vi "Main.vi"(11 "Module Admin":refnum<class "Delacor_lib_QMH_Module Admin.lvclass">) -> ()   [LabVIEW 2026, in "Servo Motor Emulator.lvlib"]
doc: "This template is based off of the Queued Message Handler design pattern and the Queued Message Handler project template that ships with LabVIEW.\n\nThe main difference is that the queue is private to this module and communication between modules is performed via Broadcast and Request events.\n\nRequest events are wrapped in public API methods and are handled in the Event Handling Loop (EHL) of this VI. Any module can register for Broadcast events sent by this module. The EHL generates messages based on user interface actions.\n\nThe Message Handling Loop (MHL) processes messages generated by the EHL, or by other messages. The messages are string values, so new messages can be added easily to the Message Cases case structure in the MHL. Each message cluster can also provide an optional value for Message Data, which is a variant that can be converted to whatever message-specific data is required.\n_____\nBased on DQMH Dev Tools: Project Template 7.1.2.1547."
uses:
  Servo Motor Emulator.lvlib
  <vilib>/Delacor/Delacor QMH/Libraries/Module Admin_class/Delacor_lib_QMH_Module Admin.lvclass
  Module Data--cluster.ctl
  Stop Argument--cluster.ctl
  <vilib>/Delacor/Delacor QMH/Libraries/Message Queue_class/Delacor_lib_QMH_Message Queue.lvclass/Delacor_lib_QMH_Message Queue.ctl
  <vilib>/Delacor/Delacor QMH/Libraries/Module Admin_class/Delacor_lib_QMH_Module Admin.lvclass/Delacor_lib_QMH_Module Admin.ctl
  Update Position Argument--cluster.ctl
  <vilib>/Utility/miscctls.llb/LVPointTypeDef.ctl
  <vilib>/Delacor/Delacor QMH/Libraries/Message Queue_class/Delacor_lib_QMH_Enqueue Message (Single).vi
  <vilib>/Delacor/Delacor QMH/Libraries/Module Admin_class/Delacor_lib_QMH_Get External Launch.vi
  <vilib>/Delacor/Delacor QMH/Libraries/Message Queue_class/Delacor_lib_QMH_Message Queue.lvclass
panel:
  in  "RH":dbl
  in  "Temperature":dbl
  out "Position":dbl(knob) scale=0.0..180.0
  out "error out":errorcluster
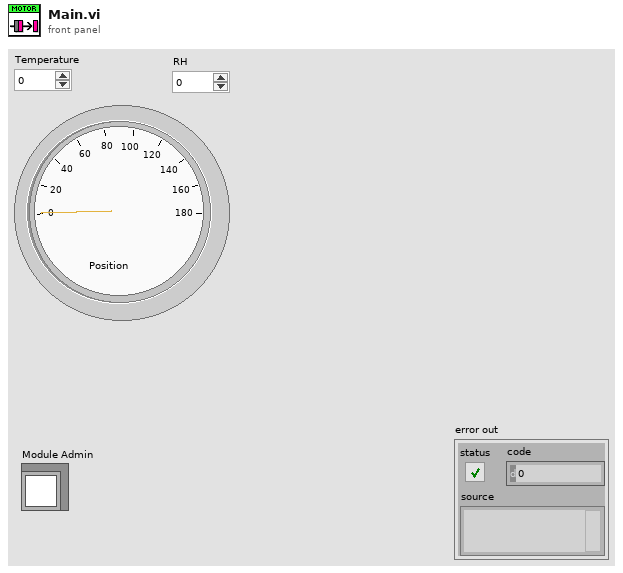
[diagram p1: front panel]
types:
  T1 = typedef "Servo Motor Emulator.lvlib/Request Events--cluster.ctl" = cluster{"Stop Module":refnum<user-event>, "Show Panel":refnum<user-event>, "Hide Panel":refnum<user-event>, "Get Module Execution Status":refnum<user-event>, "Show Diagram":refnum<user-event>, "Update Position":refnum<user-event>}
  T2 = typedef "Servo Motor Emulator.lvlib/Module Data--cluster.ctl" = cluster{"Status":string}
  T3 = enum32{"invalid lock state", "Not Locked", "Locked (No Password)", "Password-protected"}
  T4 = typedef "Servo Motor Emulator.lvlib/Stop Argument--cluster.ctl" = cluster{"Origin":string, "Exit via Stop Module Req?":bool, "Wait for Module to stop?":bool}
  T5 = typedef "Servo Motor Emulator.lvlib/Update Position Argument--cluster.ctl" = cluster{"Position":dbl}
  T6 = typedef "LVPointTypeDef.ctl" = cluster{"Horizontal":i16, "Vertical":i16}
  T7 = enum32{"Invalid", "Standard", "Closed", "Hidden", "Minimized", "Maximized"}
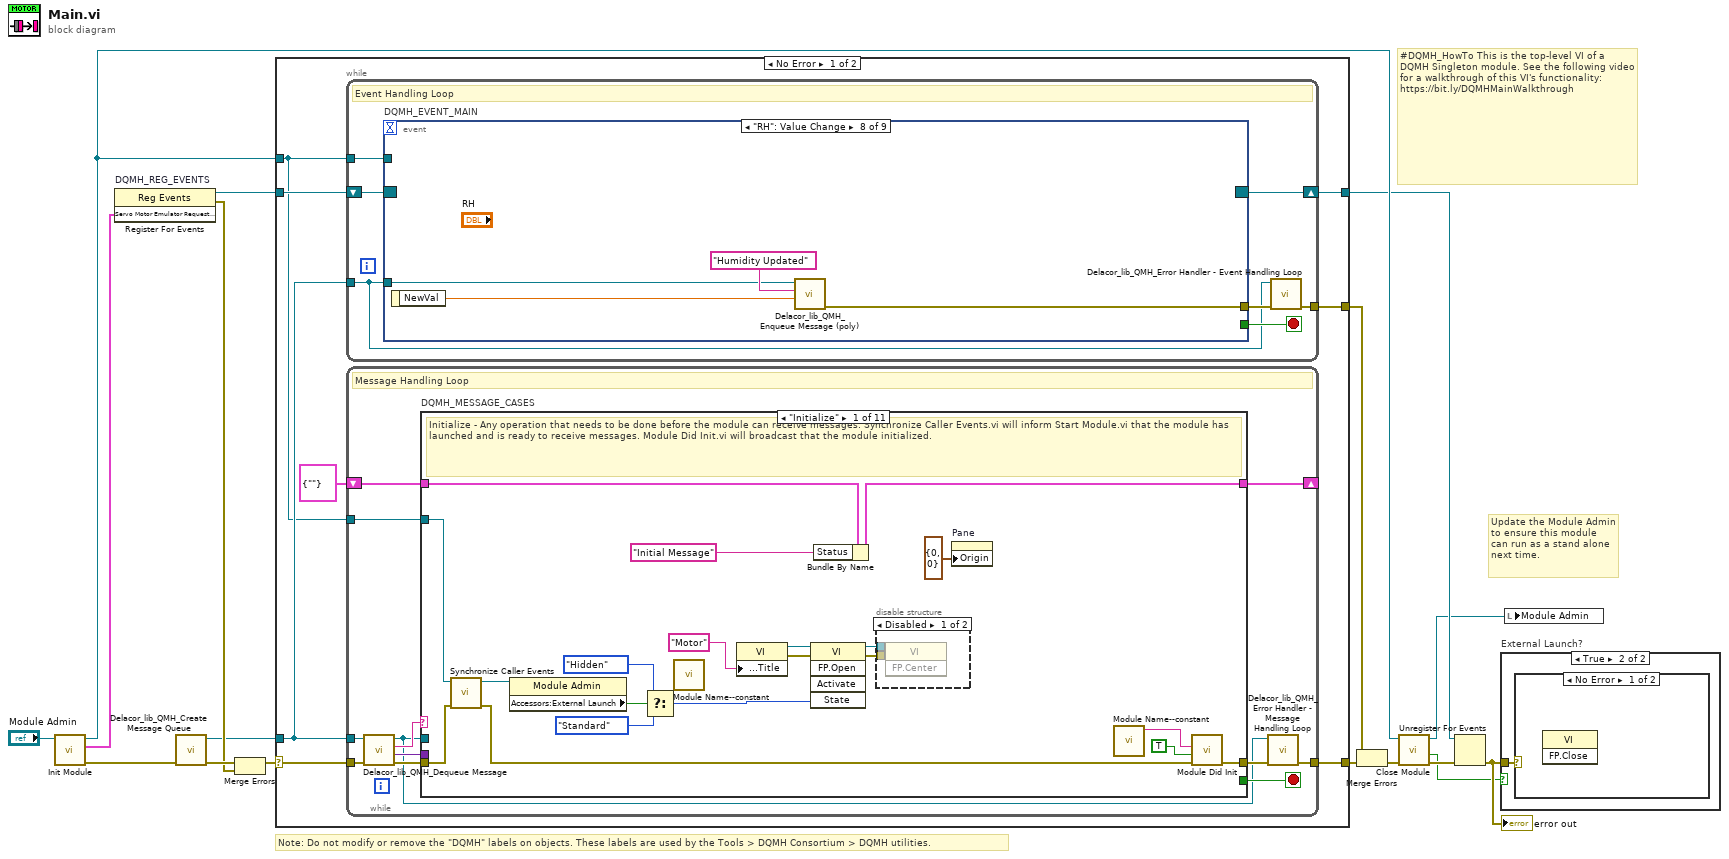
[diagram p0: block diagram]
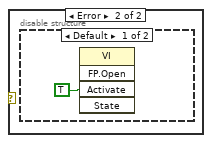
[diagram p3: hidden frame]
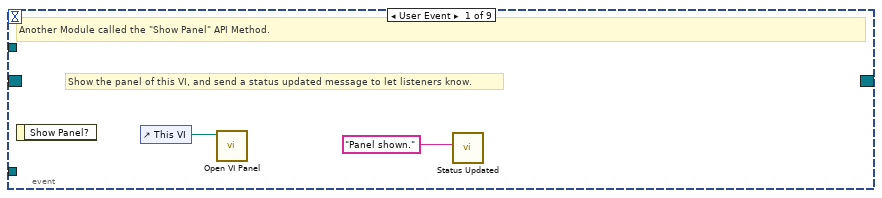
[diagram p5: hidden frame]
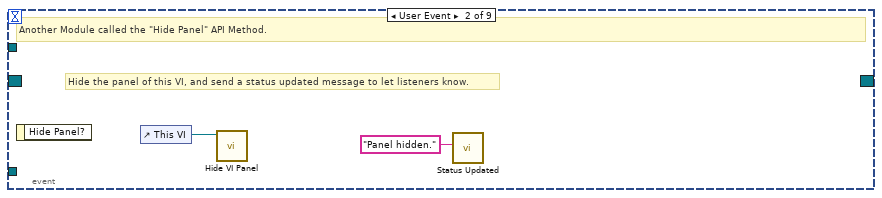
[diagram p6: hidden frame]
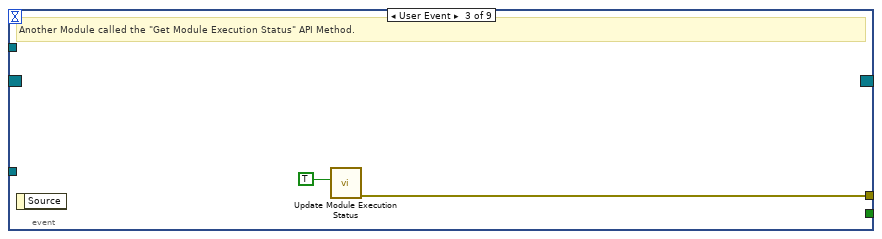
[diagram p7: hidden frame]
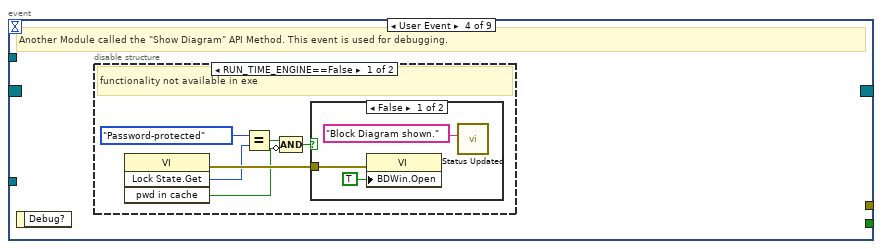
[diagram p8: hidden frame]
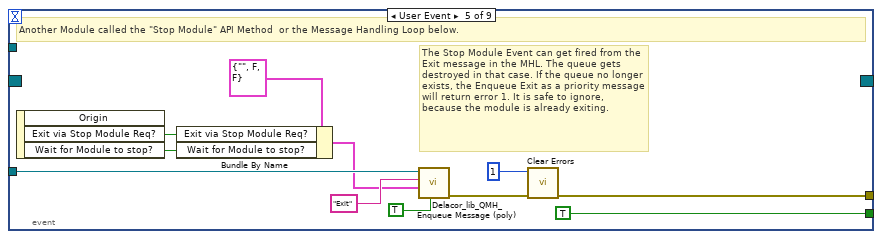
[diagram p11: hidden frame]
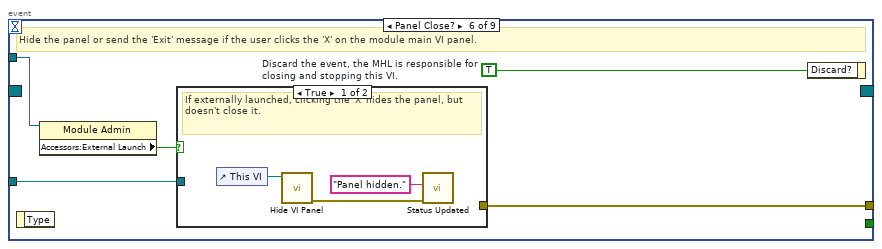
[diagram p12: hidden frame]
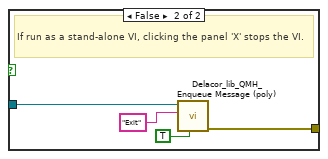
[diagram p13: hidden frame]
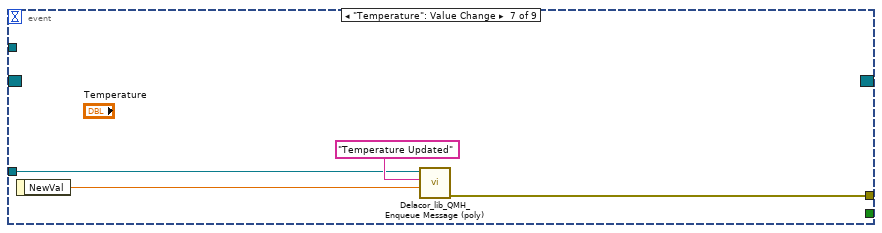
[diagram p14: hidden frame]
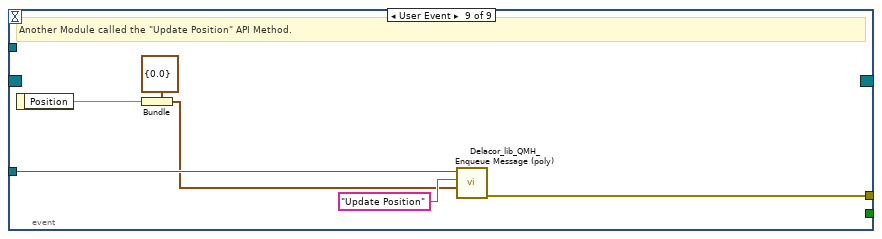
[diagram p15: hidden frame]
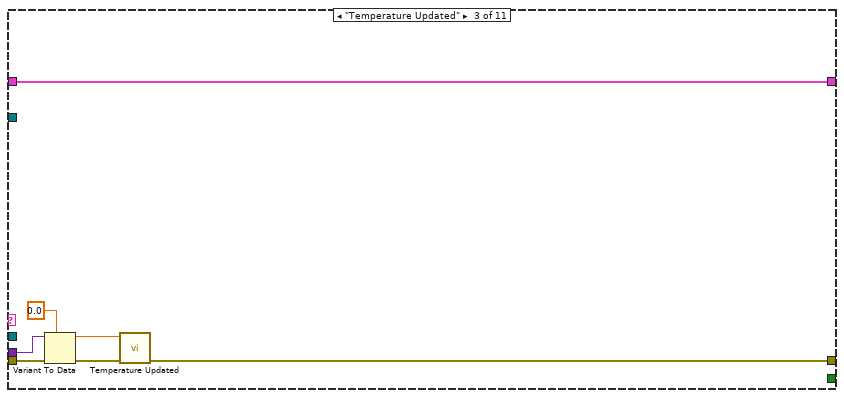
[diagram p18: hidden frame]
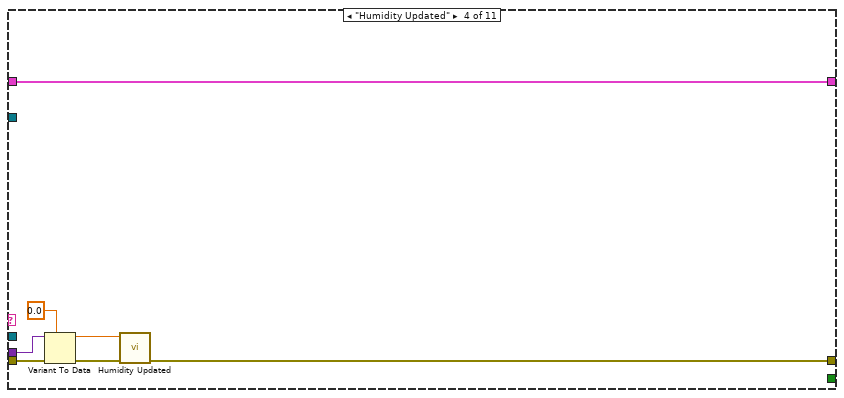
[diagram p19: hidden frame]
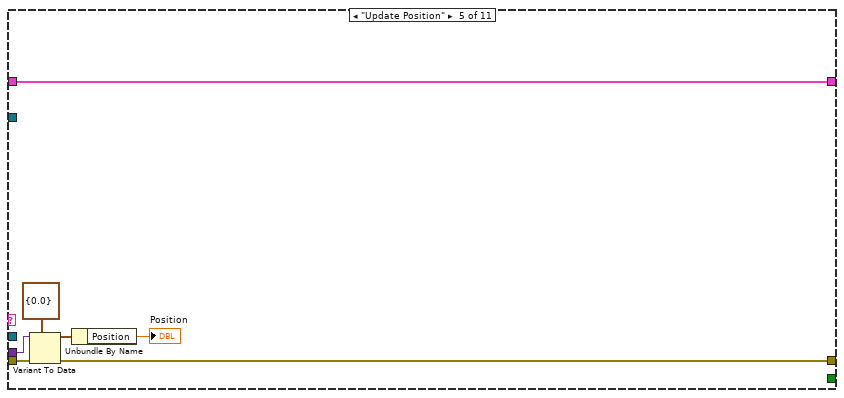
[diagram p20: hidden frame]
diagram:
  # "#DQMH_HowTo This is the top-level VI of a DQMH Singleton module. See the following video for a walkthrough of this VI's functionality: https://bit.ly/DQMHMainWalkthrough"
  # "Note: Do not modify or remove the \"DQMH\" labels on objects. These labels are used by the Tools > DQMH Consortium > DQMH utilities."
  # "Update the Module Admin to ensure this module can run as a stand alone next time."
  n1 = call "Init Module.vi"("Singleton Module Admin in"="Module Admin") -> ("error out"=w16:errorcluster, "Servo Motor Emulator Request Events"=w5:T1, "Singleton Module Admin out"=w8:refnum<class "Delacor_lib_QMH_Module Admin.lvclass">)  [unwired: 8 in]
  n2 = register-events "DQMH_REG_EVENTS"(w5) -> (reference out=w6:refnum<event-registration>, error out=w9:errorcluster)  [unwired: 2 in]
  n3 = call <vilib>:"Delacor_lib_QMH_Create Message Queue.vi"("error in"=w16) -> ("error out"=w11:errorcluster, "Message Queue"=w4:refnum<class "Delacor_lib_QMH_Message Queue.lvclass">)  [unwired: 9 in]
  n4 = Merge Errors(w11, w9) -> (w10:errorcluster)
  n5 = case shown="No Error" w10 {
    selector: w10 -> [w23 w205]
    tunnel: [w25 w204] -> w17
    tunnel: [w22 w203] -> w7
    tunnel: w6 -> [w20 w203]
    tunnel: w4 -> [w19 w198]
    tunnel: [w24 _] -> w14
    tunnel: w8 -> [w18 w199]
    frame No Error {
      n6 = while {
        tunnel: w19 -> [w26]
        shift-right: [w29] -> w22
        shift-left: w20 -> [w30]
        tunnel: [w31] -> w24
        tunnel: w18 -> [w27]
        stop <- w28 stop-if-true
        # "Event Handling Loop"
        n7 = event "DQMH_EVENT_MAIN" shown="[7] \"RH\": Value Change" {
          selector: w30 -> [_ _ _ _ _ _ _ _ _]
          dyn-events: [_ _ _ _ _ _ _ _ _] -> w29
          timeout: _ -> [_ _ _ _ _ _ _ _ _]
          tunnel: [_ _ _ _ TRUE ("Discard?") _ _ _ _] -> w28
          tunnel: w26 -> [_ _ _ _ w54 w61 w73 w77 w84]
          tunnel: [_ _ w38 _ w57 w63 w72 w76 w79] -> w32
          tunnel: w27 -> [_ _ _ _ _ w60 _ _ _]
          event User Event {
            # "Show the panel of this VI, and send a status updated message to let listeners know."
            # "Another Module called the \"Show Panel\" API Method."
            n8 = event-data() -> ()  [unwired: 1 in, 1 out]
            n9 = control-ref of="This VI"() -> (w34:refnum<vi>)
            n10 = call "Open VI Panel.vi"("VI"=w34) -> ()  [unwired: 10 in, 1 out]
            n11 = call "Status Updated.vi"("Status"="Panel shown." ("format string")) -> ()  [unwired: 10 in, 1 out]
          }
          event User Event {
            # "Hide the panel of this VI, and send a status updated message to let listeners know."
            # "Another Module called the \"Hide Panel\" API Method."
            n12 = event-data() -> ()  [unwired: 1 in, 1 out]
            n13 = control-ref of="This VI"() -> (w36:refnum<vi>)
            n14 = call "Hide VI Panel.vi"("VI"=w36) -> ()  [unwired: 10 in, 1 out]
            n15 = call "Status Updated.vi"("Status"="Panel hidden." ("format string")) -> ()  [unwired: 10 in, 1 out]
          }
          event User Event {
            # "Another Module called the \"Get Module Execution Status\" API Method."
            n16 = event-data() -> ()  [unwired: 1 in, 1 out]
            n17 = call "Update Module Execution Status.vi"("Running?"=TRUE) -> ("error out"=w38:errorcluster)  [unwired: 10 in]
          }
          event User Event {
            # "Another Module called the \"Show Diagram\" API Method. This event is used for debugging."
            n18 = event-data() -> ()  [unwired: 1 in, 1 out]
            n19 = disable-structure shown="RUN_TIME_ENGINE==False" {
              frame condition #0 (active) {
                # "functionality not available in exe"
                n20 = invoke on="Invoke Node" class="VI" method="Lock State.Get"() -> (error out=w44:errorcluster, "Get Lock State"=w43:T3, "pwd in cache"=w40:bool)  [unwired: 4 in, 1 out]
                n21 = Equal?(x=T3."Password-protected", y=w43) -> (x = y?=w41:bool)
                n22 = Compound Arithmetic op=AND(w41, invert w40) -> (w39:bool)
                n23 = case shown="False" w39 {
                  tunnel: w44 -> [w47 _]
                  frame False {
                    n24 = property on="Property Node" class="VI"(error in=w47, "BDWin.Open"=TRUE ("Block Diagram Window:Open")) -> ()  [unwired: 1 in, 2 out]
                    n25 = call "Status Updated.vi"("Status"="Block Diagram shown." ("format string")) -> ()  [unwired: 10 in, 1 out]
                  }
                  frame True {
                    # "Password-protected VI, and the password is not in the cache. Do not show the diagram."
                  }
                }
              }
              frame condition #1 {
              }
            }
          }
          event User Event {
            # "The Stop Module Event can get fired from the Exit message in the MHL. The queue gets destroyed in that case. If the queue no longer exists, the Enqueue Exit as a priority message will return error 1. It is safe to ignore, because the module is already exiting."
            # "Another Module called the \"Stop Module\" API Method  or the Message Handling Loop below."
            n26 = event-data() -> ("Exit via Stop Module Req?"=w50:bool, "Wait for Module to stop?"=w49:bool)  [unwired: 1 in, 1 out]
            n27 = Bundle By Name(cluster=T4 {"Origin"="", "Exit via Stop Module Req?"=FALSE, "Wait for Module to stop?"=FALSE} ("Stop Argument"), "Exit via Stop Module Req?"=w50, "Wait for Module to stop?"=w49) -> (w48:T4)
            n28 = call-poly <vilib>:"Delacor_lib_QMH_Enqueue Message (poly).vi"("Priority Message? (F)"=TRUE, "Message Data"=w48, "Message"="Exit", "Message Queue in"=w54) -> ("error out"=w58:errorcluster)  [unwired: 6 in, 1 out]
            n29 = call <vilib>:"Clear Errors.vi"("error in (no error)"=w58, "specific error code to clear (0: all)"=1) -> ("error out"=w57:errorcluster)  [unwired: 4 in, 1 out]
          }
          event Panel Close? {
            w62 = TRUE  # Discard the event, the MHL is responsible for closing and stopping this VI.
            # "Hide the panel or send the 'Exit' message if the user clicks the 'X' on the module main VI panel."
            n30 = event-data() -> ()  [unwired: 1 in, 1 out]
            n31 = property on="Property Node" class="Module Admin"(reference=w60) -> ("Accessors:External Launch"=w59:bool)  [unwired: 1 in, 2 out]
            n32 = case shown="True" w59 {
              tunnel: w61 -> [_ w69]
              tunnel: [_ w70] -> w63
              frame True {
                # "If externally launched, clicking the 'X' hides the panel, but doesn't close it."
                n33 = control-ref of="This VI"() -> (w66:refnum<vi>)
                n34 = call "Hide VI Panel.vi"("VI"=w66) -> ("error out"=w64:errorcluster)  [unwired: 10 in]
                n35 = call "Status Updated.vi"("error in"=w64, "Status"="Panel hidden." ("format string")) -> ()  [unwired: 9 in, 1 out]
              }
              frame False {
                # "If run as a stand-alone VI, clicking the panel 'X' stops the VI."
                n36 = call-poly <vilib>:"Delacor_lib_QMH_Enqueue Message (poly).vi"("Priority Message? (F)"=TRUE, "Message"="Exit", "Message Queue in"=w69) -> ("error out"=w70:errorcluster)  [unwired: 7 in, 1 out]
              }
            }
            n37 = event-data ("Event Filter Node")("Discard?"=w62) -> ()  [unwired: 1 in, 1 out]
          }
          event "Temperature": Value Change {
            n38 = event-data() -> ("NewVal"=w71:dbl)  [unwired: 1 in]
            n39 = call-poly <vilib>:"Delacor_lib_QMH_Enqueue Message (poly).vi"("Message Data"=w71, "Message"="Temperature Updated", "Message Queue in"=w73) -> ("error out"=w72:errorcluster)  [unwired: 7 in, 1 out]
          }
          event "RH": Value Change {
            n40 = event-data() -> ("NewVal"=w75:dbl)  [unwired: 1 in]
            n41 = call-poly <vilib>:"Delacor_lib_QMH_Enqueue Message (poly).vi"("Message Data"=w75, "Message"="Humidity Updated", "Message Queue in"=w77) -> ("error out"=w76:errorcluster)  [unwired: 7 in, 1 out]
          }
          event User Event {
            # "Another Module called the \"Update Position\" API Method."
            n42 = event-data() -> ("Position"=w80:dbl)  [unwired: 1 in]
            n43 = Bundle(cluster=T5 {"Position"=0.0} ("Update Position Argument"), "Position"=w80) -> (w81:T5)
            n44 = call-poly <vilib>:"Delacor_lib_QMH_Enqueue Message (poly).vi"("Message Data"=w81, "Message"="Update Position", "Message Queue in"=w84) -> ("error out"=w79:errorcluster)  [unwired: 7 in, 1 out]
          }
        }
        n45 = call-dynamic "Delacor_lib_QMH_Error Handler - Event Handling Loop.vi"("error in"=w32, "Message Queue in"=w26) -> ("dup error in"=w31:errorcluster)  [unwired: 8 in, 1 out]
      }
      n46 = while {
        tunnel: w19 -> [w85]
        shift-right: [w93] -> _
        shift-left: T2 {"Status"=""} ("Data Cluster") -> [w94]
        tunnel: w23 -> [w96]
        tunnel: [w88] -> w25
        tunnel: w18 -> [w89]
        stop <- w92 stop-if-true
        # "Message Handling Loop"
        n47 = call-dynamic "Delacor_lib_QMH_Dequeue Message.vi"("error in"=w96, "Message Queue in"=w85) -> ("error out"=w95:errorcluster, "Message Data"=w90:variant, "Message"=w91:string, "Message Queue out"=w86:refnum<class "Delacor_lib_QMH_Message Queue.lvclass">)  [unwired: 6 in]
        n48 = case "DQMH_MESSAGE_CASES" shown="\"Initialize\"" w91 {
          selector: w91 -> [_ _ _ _ _ _ _ _ _ _ w193]
          tunnel: w86 -> [_ _ _ _ _ _ _ _ w159 w181 _]
          tunnel: w95 -> [w114 w120 w122 w129 w141 w144 w146 w155 w166 w187 w196]
          tunnel: [w112 w120 w123 w130 w139 w143 w146 w154 w162 w182 w197] -> w87
          tunnel: w94 -> [w104 w119 w127 w134 w140 w142 w145 w152 w161 w180 w194]
          tunnel: [w103 w119 w127 w134 w140 w142 w145 w152 w161 w180 w194] -> w93
          tunnel: [_ _ _ _ _ _ _ _ _ w179 _] -> w92
          tunnel: w90 -> [_ _ w126 w133 w138 _ _ _ w160 w178 _]
          tunnel: w89 -> [w105 _ _ _ _ _ _ _ w158 w173 _]
          frame "Initialize" {
            # "Initialize - Any operation that needs to be done before the module can receive messages. Synchronize Caller Events.vi will inform Start Module.vi that the module has launched and is ready to receive messages. Module Did Init.vi will broadcast that the module initialized."
            n49 = call "Synchronize Caller Events.vi"("error in"=w114, "Singleton Module Admin in"=w105) -> ("error out"=w113:errorcluster, "Singleton Module Admin out"=w100:refnum<class "Delacor_lib_QMH_Module Admin.lvclass">)  [unwired: 8 in]
            n50 = property on="Property Node" class="Module Admin"(reference=w100) -> ("Accessors:External Launch"=w109:bool)  [unwired: 1 in, 2 out]
            n51 = Select(t=T7."Hidden" ("State"), s=w109, f=T7."Standard" ("State")) -> (s? t:f=w106:T7)
            n52 = call "Module Name--constant.vi"() -> ()  [unwired: 11 in, 1 out]
            n53 = property on="Property Node" class="VI"("Front Panel.Title"="Motor" ("Front Panel Window:Title")) -> (reference out=w111:refnum<vi>, error out=w116:errorcluster)  [unwired: 2 in]
            n54 = invoke on="Invoke Node" class="VI" method="FP.Open"(reference=w111, error in=w116, "State"=w106) -> (reference out=w110:refnum<vi>, error out=w115:errorcluster)  [unwired: 2 in, 3 out]
            n55 = Bundle By Name(cluster=w104, "Status"="Initial Message" ("Initial Message")) -> (w103:T2)
            n56 = disable-structure shown="Disabled" {
              disable-tunnel: w115 -> [w118 _]
              disable-tunnel: w110 -> [w117 _]
              frame Disabled {
                n57 = invoke on="Invoke Node" class="VI" method="FP.Center"(reference=w117, error in=w118) -> ()  [unwired: 1 in, 3 out]
              }
              frame Enabled {
              }
            }
            n58 = property on="Pane" class="Pane"("Origin"=T6 {"Horizontal"=0, "Vertical"=0}) -> ()  [unwired: 2 in, 2 out]
            n59 = call "Module Name--constant.vi"() -> ("Module Name"=w101:string)  [unwired: 11 in]
            n60 = call "Module Did Init.vi"("error in"=w113, "Initialized?"=TRUE, "Origin"=w101) -> ("error out"=w112:errorcluster)  [unwired: 8 in]
          }
          frame "---Module Specific---" {
            # "Separator -- The following cases handle messages specific to this Module."
          }
          frame "Temperature Updated" {
            n61 = Variant To Data(error in=w122, type=0.0 ("Temperature"), Variant=w126) -> (data=w124:dbl, error out=w121:errorcluster)
            n62 = call "Temperature Updated.vi"("error in"=w121, "Temperature"=w124) -> ("error out"=w123:errorcluster)  [unwired: 9 in]
          }
          frame "Humidity Updated" {
            n63 = Variant To Data(error in=w129, type=0.0 ("Temperature"), Variant=w133) -> (data=w131:dbl, error out=w128:errorcluster)
            n64 = call "Humidity Updated.vi"("error in"=w128, "Humidity"=w131) -> ("error out"=w130:errorcluster)  [unwired: 9 in]
          }
          frame "Update Position" {
            n65 = Variant To Data(error in=w141, type=T5 {"Position"=0.0} ("Update Position Argument"), Variant=w138) -> (data=w136:T5, error out=w139:errorcluster)
            n66 = Unbundle By Name(w136) -> ("Position"=→"Position":dbl)
          }
          frame "---Copy This Frame---" {
            # "Duplicate this frame when creating new messages.  Change this comment in the duplicated frame to describe this message."
            n67 = Merge Errors(w144) -> (w143:errorcluster)
          }
          frame "---Exit and Error Handling---" {
            # "Separator - The following cases handle errors and exit messages."
          }
          frame "Simulate MHL Error" {
            # "#DQMH_HowTo The 'Simulate MHL Error' button  illustrates how the MHL handles errors. This event is instructional in nature and can be removed."
            # "Simulate an error occurring at the MHL"
            n68 = call "Module Name--constant.vi"() -> ("Module Name"=w148:string)  [unwired: 11 in]
            n69 = Format Into String(format string="Simulated error originating at Message Handling Loop in %s", w148) -> (resulting string=w149:string)  [unwired: 2 in, 1 out]
            n70 = call <vilib>:"Error Cluster From Error Code.vi"("show call chain? (False)"=TRUE, "error message (\"\")"=w149, "error code (0)"=5001) -> ("error out"=w153:errorcluster)  [unwired: 6 in]
            n71 = Merge Errors(w155, w153) -> (w154:errorcluster)
          }
          frame "Error" {
            # "#DQMH_CodeRecommended - If the module is running in standalone mode (External Launch = FALSE), this code will pop up an error dialog and call the 'Exit' message if an error occurs. Add more fine-grained error management here."
            # "Error - Check the error message data and respond accordingly. This message is sent by the \"Error Handler\" VIs at the end of each loop in this application."
            n72 = property on="Property Node" class="Module Admin"(reference=w158) -> ("Accessors:External Launch"=w157:bool)  [unwired: 1 in, 2 out]
            n73 = Variant To Data(error in=w166, type=errorcluster {"status"=FALSE, "code"=0, "source"=""} ("error constant"), Variant=w160) -> (data=w156:errorcluster, error out=w164:errorcluster)
            n74 = local write "error out"(w156) -> ()
            n75 = call "Error Reported.vi"("Error"=w156) -> ()  [unwired: 10 in, 1 out]
            n76 = case shown="False" w157 {
              tunnel: [w171 _] -> w163
              tunnel: w159 -> [w169 _]
              tunnel: w156 -> [w170 _]
              frame False {
                n77 = disable-structure shown="Default" {
                  disable-tunnel: w170 -> [w172 _]
                  frame condition #0 (active) {
                    # "If the module is running standalone, then pop up an error dialog and call the \"Exit\" message."
                    n78 = call <vilib>:"Simple Error Handler.vi"("error in (no error)"=w172) -> ()  [unwired: 4 in, 5 out]
                  }
                  frame condition #1 {
                    # "To prevent the Simple Error Handler VI from being loaded (e.g. when deploying to a Real-Time target), add the Conditional Disable Symbol \"DQMH_Disable_SEH\" to your project and set it to TRUE."
                  }
                }
                n79 = call-poly <vilib>:"Delacor_lib_QMH_Enqueue Message (poly).vi"("Priority Message? (F)"=TRUE, "Message"="Exit", "Message Queue in"=w169) -> ("error out"=w171:errorcluster)  [unwired: 7 in, 1 out]
              }
              frame True {
                # "If the module was launched externally, calling the Error Reported broadcast VI is the only action performed by the \"Error\" message. The module's caller can then process the error appropriately."
              }
            }
            n80 = Merge Errors(w164, w163) -> (w162:errorcluster)
          }
          frame "Exit" {
            w177 = 91  # 91: not all Exit messages will have an argument
            w179 = TRUE  # Stop the VI
            # "Release the message queue reference"
            # "#DQMH_CodeNeeded - Add any required cleanup code here."
            # "Exit - Exit the application."
            n81 = Variant To Data(error in=w187, type=T4 {"Origin"="", "Exit via Stop Module Req?"=FALSE, "Wait for Module to stop?"=FALSE} ("Stop Argument"), Variant=w178) -> (data=w175:T4, error out=w184:errorcluster)
            n82 = call <vilib>:"Clear Errors.vi"("error in (no error)"=w184, "specific error code to clear (0: all)"=w177) -> ("error out"=w186:errorcluster)  [unwired: 4 in, 1 out]
            n83 = control-ref of="This VI"() -> (w174:refnum<vi>)
            n84 = call-dynamic "Delacor_lib_QMH_Release Message Queue.vi"("error in"=w186, "Message Queue"=w181) -> ("error out"=w185:errorcluster)  [unwired: 9 in]
            n85 = call "Handle Exit.vi"("Stop Argument"=w175, "Admin in"=w173, "VI reference"=w174) -> ("error out"=w183:errorcluster)  [unwired: 7 in, 1 out]
            n86 = Merge Errors(w185, w183) -> (w182:errorcluster)
            n87 = call "Error Reported.vi"("Error"=w182) -> ()  [unwired: 10 in, 1 out]
          }
          frame Default {
            # "'Default' case only runs if there is a message that isn't defined in any of the other cases.  Output a programming error."
            n88 = call "Module Name--constant.vi"() -> ("Module Name"=w192:string)  [unwired: 11 in]
            n89 = Format Into String(format string="The invalid message string \"%s\" was received in the Message Handling Loop for module \"%s\".", w193, w192) -> (resulting string=w188:string)  [unwired: 2 in, 1 out]
            n90 = call <vilib>:"Error Cluster From Error Code.vi"("show call chain? (False)"=TRUE, "error message (\"\")"=w188, "error code (0)"=1) -> ("error out"=w195:errorcluster)  [unwired: 6 in]
            n91 = Merge Errors(w196, w195) -> (w197:errorcluster)
          }
        }
        n92 = call-dynamic "Delacor_lib_QMH_Error Handler - Message Handling Loop.vi"("error in"=w87, "Message Queue in"=w86) -> ("dup error in"=w88:errorcluster)  [unwired: 8 in, 1 out]
      }
    }
    frame Error {
      # "Synchronize Caller Events.vi will inform Start Module.vi that the module has launched and will let the code calling Start Module.vi register for broadcasts and would permit the caller receive the broadcast that an error occurred at launch time."
      n93 = call-dynamic "Delacor_lib_QMH_Release Message Queue.vi"("error in"=w205, "Message Queue"=w198) -> ("error out"=w204:errorcluster)  [unwired: 9 in]
      n94 = call "Synchronize Caller Events.vi"("Singleton Module Admin in"=w199) -> ("error out"=w206:errorcluster)  [unwired: 9 in, 1 out]
      n95 = call "Module Name--constant.vi"() -> ("Module Name"=w202:string)  [unwired: 11 in]
      n96 = Format Into String(format string="An error occurred during initialization. %s is no longer running.", w202) -> (resulting string=w200:string)  [unwired: 2 in, 1 out]
      n97 = Merge Errors(w204, w206) -> (w207:errorcluster)
      n98 = call "Error Reported.vi"("Additional Information"=w200, "Error"=w207) -> ()  [unwired: 9 in, 1 out]
    }
  }
  n99 = Merge Errors(w14, w17) -> (w13:errorcluster)
  n100 = call "Close Module.vi"("error in"=w13, "Module Admin in"=w8) -> ("error out"=w15:errorcluster, "External Launch"=w1:bool, "Module Admin out"=w2:refnum<class "Delacor_lib_QMH_Module Admin.lvclass">)  [unwired: 7 in]
  n101 = Unregister For Events(event registration refnum=w7, error in=w15) -> (error out=w12:errorcluster)
  "error out" <- w12
  n102 = case "External Launch?" shown="True" w1 {
    tunnel: w12 -> [_ w208]
    frame False {
    }
    frame True {
      n103 = case shown="No Error" w208 {
        frame No Error {
          n104 = invoke on="Invoke Node" class="VI" method="FP.Close"() -> ()  [unwired: 3 in, 3 out]
        }
        frame Error {
          n105 = disable-structure shown="Default" {
            frame condition #0 (active) {
              n106 = invoke class="VI" method="FP.Open"("Activate"=TRUE ("Activate?")) -> ()  [unwired: 4 in, 5 out]
            }
            frame condition #1 {
              # "Don't show panel on error if running inside a built EXE."
            }
          }
        }
      }
    }
  }
  n107 = local write "Module Admin"(w2) -> ()
